vi "count_string_matches.vi"() -> ()   [LabVIEW 2014]
doc: "This VI shows two different ways to count how many times a character occurs within a string. In the first way, LabVIEW converts the string to a byte array and then indexes through each byte using a For Loop. LabVIEW compares each byte to the *. In the second way, LabVIEW uses a While Loop to iteratively parse through the incoming string. The example uses * as the character to search for."
panel:
  out "Number of matches 2":i32=7
  in  "String 2":string="h*el*l*o**w*or*ld"
  out "Number of matches 1":i32=7
  in  "String 1":string="h*el*l*o**w*or*ld"
  # "Select Help»Show Context Help and move the cursor over the VI icon to display help for this VI."
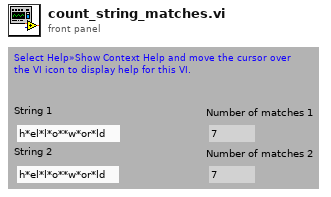
[diagram p1: front panel]
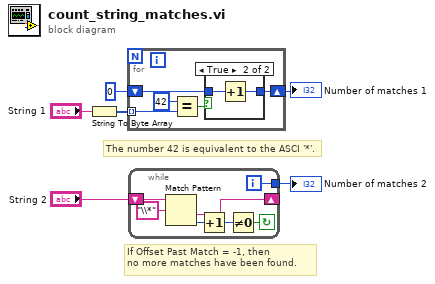
[diagram p0: block diagram]
diagram:
  # "If Offset Past Match = -1, then\nno more matches have been found."
  # "The number 42 is equivalent to the ASCI '*'."
  n1 = String To Byte Array(string="String 1") -> (unsigned byte array=w3:u8[])
  n2 = for {
    shift-right: [w9] -> w5
    shift-left: 0 -> [w10]
    tunnel: w3 -> [w8] mode=indexing
    n3 = Equal?(x=u8 42, y=w8) -> (x = y?=w11:bool)
    n4 = case shown="True" w11 {
      tunnel: w10 -> [w12 w14]
      tunnel: [w12 w13] -> w9
      frame False {
      }
      frame True {
        n5 = Increment(x=w14) -> (x+1=w13:i32)
      }
    }
  }
  "Number of matches 1" <- w5
  n6 = while {
    tunnel: [w15] -> w1
    shift-left: "String 2" -> [w21]
    shift-right: [w19] -> _
    i -> [w15]
    stop <- w16 continue-if-true
    n7 = Match Pattern(string=w21, regular expression="\\*") -> (after substring=w19:string, offset past match=w18:i32)  [unwired: 1 in, 2 out]
    n8 = Increment(x=w18) -> (x+1=w17:i32)
    n9 = Not Equal To 0?(x=w17) -> (x != 0?=w16:bool)
  }
  "Number of matches 2" <- w1
